vi "Read Value Without Comment.vi"(7 "section":string, 8 "error in (no error)":errorcluster, 10 "key":string, 11 "refnum":T1) -> (0 "error out":errorcluster, 1 "value":string, 2 "found?":bool, 3 "refnum out":T1)   [LabVIEW 2020, in "NI_LVConfig.lvlib"]
uses:
  <vilib>/Utility/config.llb/NI_LVConfig.lvlib
  <vilib>/Utility/config.llb/Config Data RefNum.ctl
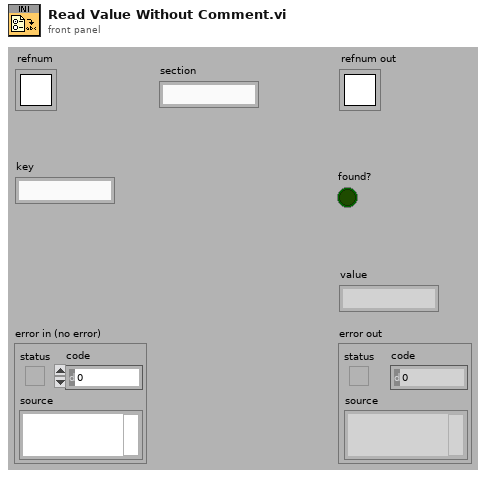
[diagram p1: front panel]
types:
  T1 = typedef "NI_LVConfig.lvlib/Config Data RefNum.ctl" = refnum<k1>
  T2 = typedef "NI_LVConfig.lvlib/Config Queue.ctl" = refnum<queue>
  T3 = typedef "NI_LVConfig.lvlib/Config Data.ctl" = cluster{"sections":T4[], "path":path, "dirty":bool}
  T4 = typedef "NI_LVConfig.lvlib/Section.ctl" = cluster{"name":string, "comment":string, "kvc":string[][]}
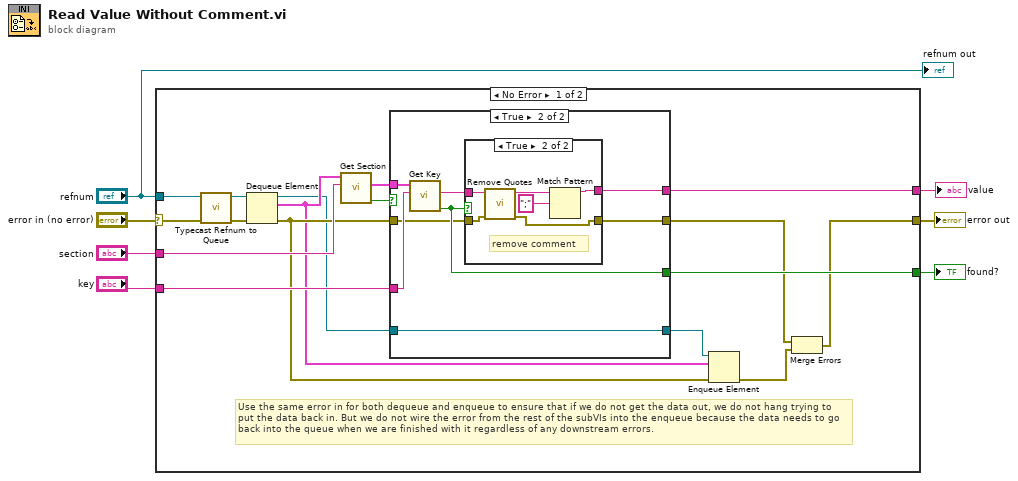
[diagram p0: block diagram]
diagram:
  n1 = case shown="No Error" "error in (no error)" {
    selector: "error in (no error)" -> [w20 w41]
    tunnel: [w8 w41] -> w6
    tunnel: "refnum" -> [w22 _]
    tunnel: "section" -> [w19 _]
    tunnel: "key" -> [w16 _]
    tunnel: [w23 _] -> w3
    tunnel: [w15 _] -> w1
    frame No Error {
      # "Use the same error in for both dequeue and enqueue to ensure that if we do not get the data out, we do not hang trying to put the data back in. But we do not wire the error from the rest of the subVIs into the enqueue because the data needs to go back into the queue when we are finished with it regardless of any downstream errors."
      n2 = call <vilib>:"Typecast Refnum to Queue.vi"("refnum in"=w22) -> ("queue out"=w21:T2)  [unwired: 10 in]
      n3 = Dequeue Element(queue=w21, error in (no error)=w20) -> (queue out=w11:T2, element=w13:T3, error out=w14:errorcluster)  [unwired: 1 in, 1 out]
      n4 = call <vilib>:"Get Section.vi"("section"=w19, "element"=w13) -> ("section exists?"=w18:bool, "section data"=w17:T4)  [unwired: 6 in, 2 out]
      n5 = case shown="True" w18 {
        tunnel: [_ w33] -> w23
        tunnel: [w25 w32] -> w10
        tunnel: w17 -> [_ w31]
        tunnel: w16 -> [_ w30]
        tunnel: [_ w28] -> w15
        tunnel: w14 -> [w25 w27]
        tunnel: [w24 w26] -> w12
        tunnel: w11 -> [w24 w26]
        frame False {
        }
        frame True {
          n6 = call <vilib>:"Get Key.vi"("key"=w30, "section data"=w31) -> ("key exists?"=w28:bool, "value"=w29:string)  [unwired: 5 in, 3 out]
          n7 = case shown="True" w28 {
            tunnel: [_ w37] -> w33
            tunnel: [w34 w35] -> w32
            tunnel: w29 -> [_ w38]
            tunnel: w27 -> [w34 w36]
            frame False {
            }
            frame True {
              # "remove comment"
              n8 = call <vilib>:"Remove Quotes.vi"("error in (no error)"=w36, "string"=w38) -> ("error out"=w35:errorcluster, "without quotes"=w39:string)  [unwired: 7 in, 1 out]
              n9 = Match Pattern(string=w39, regular expression=";") -> (before substring=w37:string)  [unwired: 1 in, 3 out]
            }
          }
        }
      }
      n10 = Enqueue Element(queue=w12, element=w13, error in (no error)=w14) -> (error out=w9:errorcluster)  [unwired: 1 in, 2 out]
      n11 = Merge Errors(w10, w9) -> (w8:errorcluster)
    }
    frame Error {
    }
  }
  "error out" <- w6
  "found?" <- w1
  "value" <- w3
  "refnum out" <- "refnum"
